vi "Bind Delete Command Parameters.vi"(8 "Error In (no error)":errorcluster, 10 "Record":variant, 11 "SQL Statement In":refnum<class "SQL Statement.lvclass">) -> (0 "Error Out":errorcluster, 3 "SQL Statement Out":refnum<class "SQL Statement.lvclass">)   [LabVIEW 2023, in "SQLite DB Operator.lvclass"]
uses:
  <vilib>/drjdpowell/SQLite Library/SQL Statement/SQL Statement.lvclass
  DB Records/Expenses Tracker Balance/Public/Ctrls/Balance.ctl
  <vilib>/drjdpowell/SQLite Library/SQL Statement/SQL Statement.lvclass/SQL Statement.ctl
  DB Records/Expenses Tracker Category/Public/Ctrls/Category.ctl
  DB Records/Expenses Tracker Cycle/Public/Ctrls/Cycle.ctl
  DB Records/Expenses Tracker Saving Goal/Public/Ctrls/Saving Goal.ctl
  DB Records/Expenses Tracker Saving/Public/Ctrls/Saving.ctl
  DB Records/Expenses Tracker Subcategory/Public/Ctrls/Subcategory.ctl
  DB Records/Expenses Tracker Transaction/Public/Ctrls/Transaction.ctl
  <vilib>/drjdpowell/SQLite Library/SQL Statement/Bind Null.vi
  <vilib>/drjdpowell/SQLite Library/SQL Statement/Bind Timestamp (Real).vi
  <vilib>/drjdpowell/SQLite Library/SQL Statement/Bind Real.vi
  <vilib>/drjdpowell/SQLite Library/SQL Statement/Bind Integer.vi
  <vilib>/drjdpowell/SQLite Library/SQL Statement/Bind Text.vi
  <vilib>/drjdpowell/SQLite Library/SQL Statement/Error Message.vi
  SQLite DB Operator.lvclass
  SQLite DB Operator.lvclass/SQLite DB Operator.ctl
  DB Records/Expenses Tracker Category/Expenses Tracker Category.lvclass
  <vilib>/Utility/Data Type/NI_Data Type.lvlib
  DB Records/Expenses Tracker Transaction/Expenses Tracker Transaction.lvclass
  DB Records/Expenses Tracker Subcategory/Expenses Tracker Subcategory.lvclass
  DB Records/Expenses Tracker Balance/Expenses Tracker Balance.lvclass
  DB Records/Expenses Tracker Cycle/Expenses Tracker Cycle.lvclass
  DB Records/Expenses Tracker Saving Goal/Expenses Tracker Saving Goal.lvclass
  DB Records/Expenses Tracker Saving/Expenses Tracker Saving.lvclass
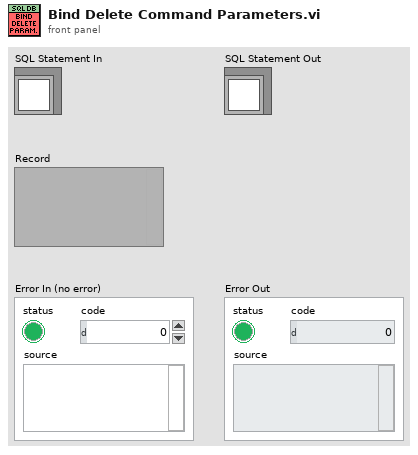
[diagram p1: front panel]
types:
  T1 = typedef "Expenses Tracker Balance.lvclass/Balance.ctl" = cluster{"ID":u8, "Value":dbl, "Last_update":timestamp}
  T2 = typedef "Expenses Tracker Category.lvclass/Category.ctl" = cluster{"ID":u32, "Name":string}
  T3 = typedef "Expenses Tracker Cycle.lvclass/Cycle.ctl" = cluster{"ID":u32, "Name":string, "Day_of_occurence":u8, "Description":string}
  T4 = typedef "Expenses Tracker Saving Goal.lvclass/Saving Goal.ctl" = cluster{"ID":u32, "Name":string, "Current_value":dbl, "Target_value":dbl, "Date_of_entry":timestamp, "Due_date":timestamp, "Last_update":timestamp, "Description":string}
  T5 = typedef "Expenses Tracker Saving.lvclass/Saving.ctl" = cluster{"ID":u32, "Saving_goal":u32, "Value":dbl, "Date_of_entry":timestamp, "Description":string}
  T6 = typedef "Expenses Tracker Subcategory.lvclass/Subcategory.ctl" = cluster{"ID":u32, "Name":string, "Category":u32}
  T7 = typedef "Expenses Tracker Transaction.lvclass/Transaction.ctl" = cluster{"ID":u32, "Name":string, "Is_income":bool, "Value":dbl, "Amount":dbl, "Total":dbl, "Date_of_entry":timestamp, "Date_of_occurence":timestamp, "Last_update":timestamp, "Category":u32, "Subcategory":u32, "Cycle":u32, "Description":string}
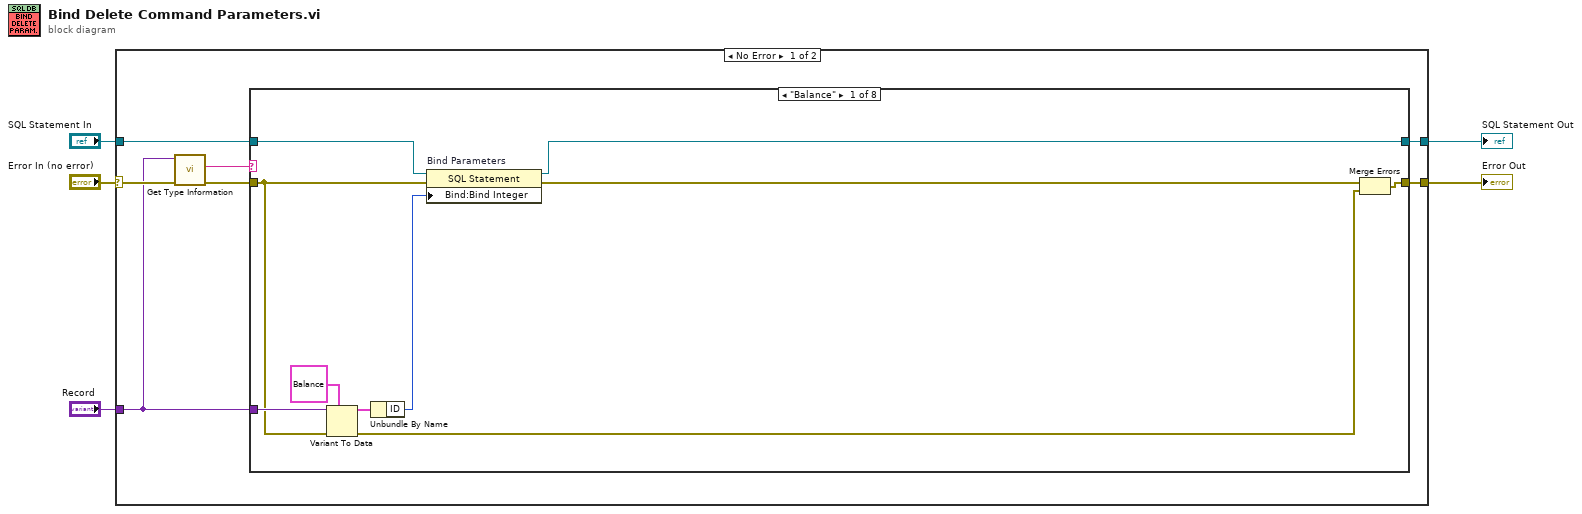
[diagram p0: block diagram]
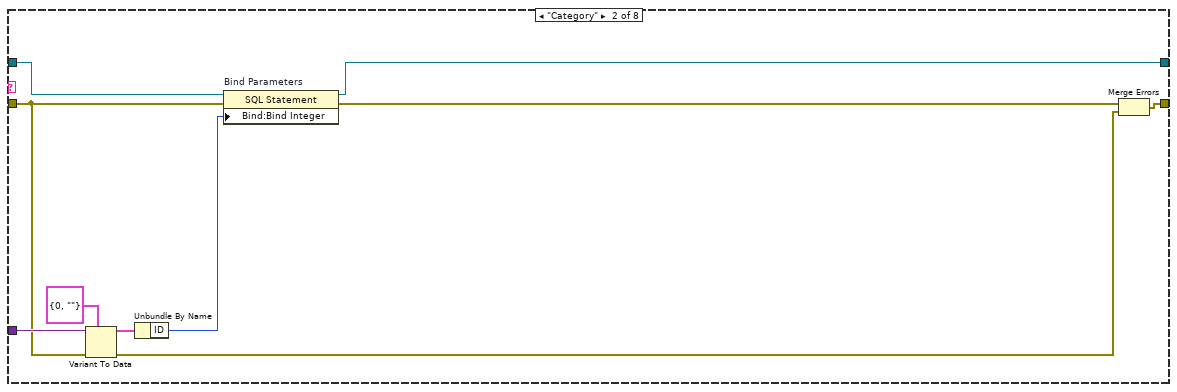
[diagram p2: hidden frame]
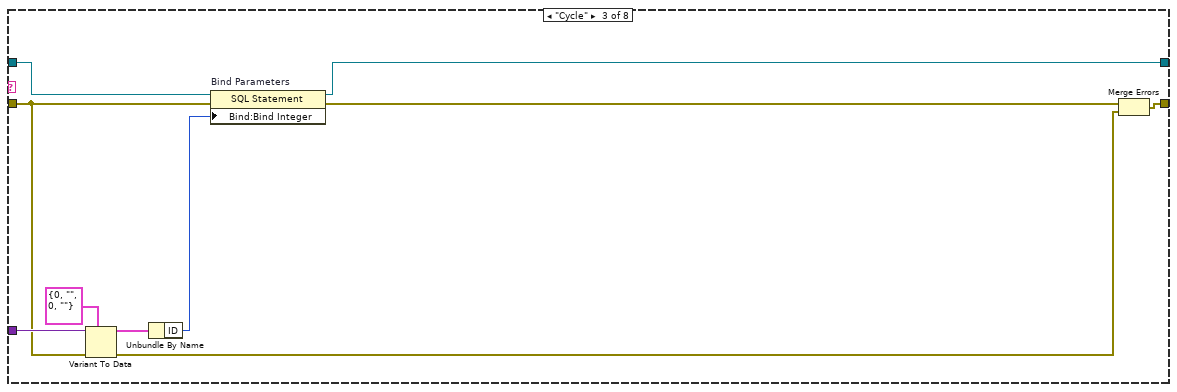
[diagram p3: hidden frame]
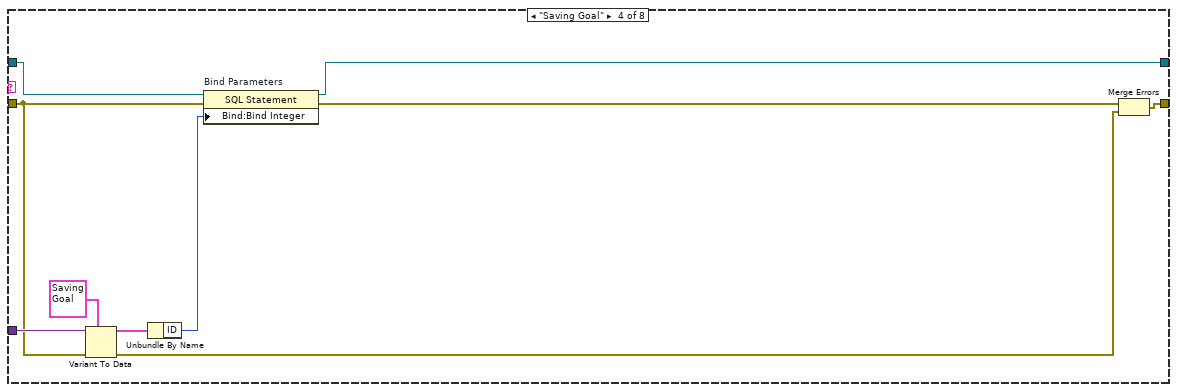
[diagram p4: hidden frame]
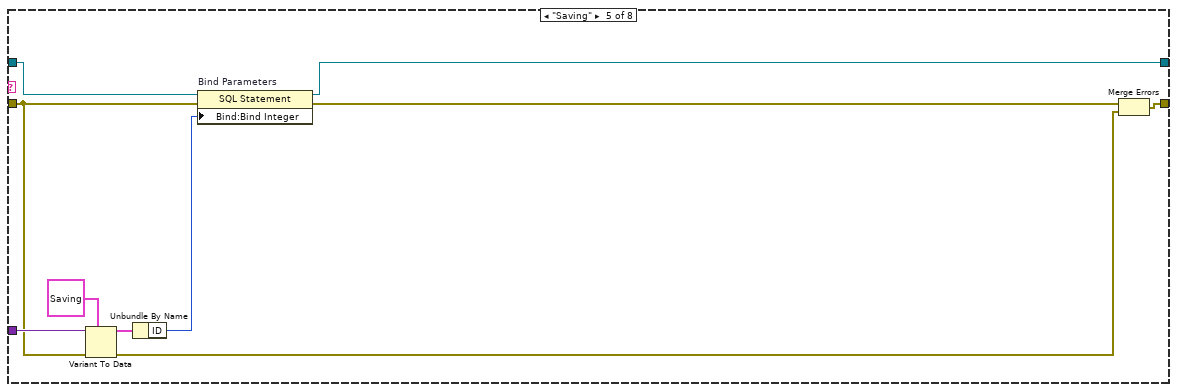
[diagram p5: hidden frame]
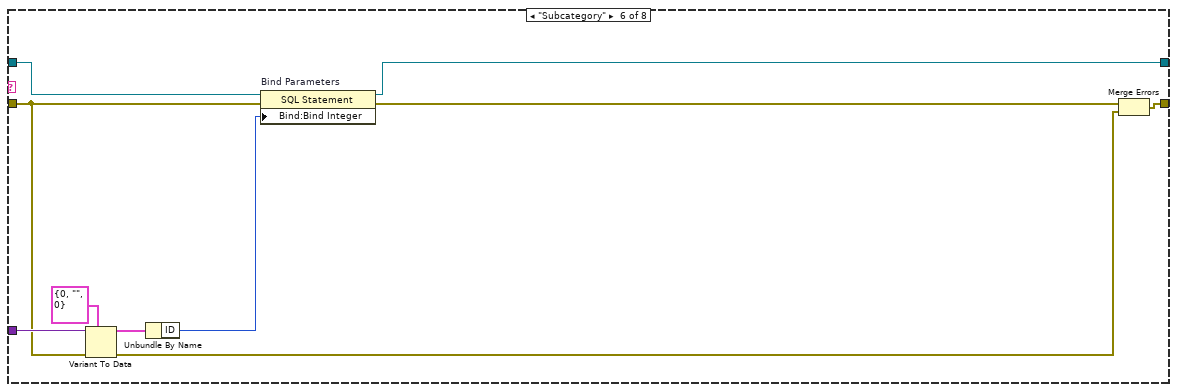
[diagram p6: hidden frame]
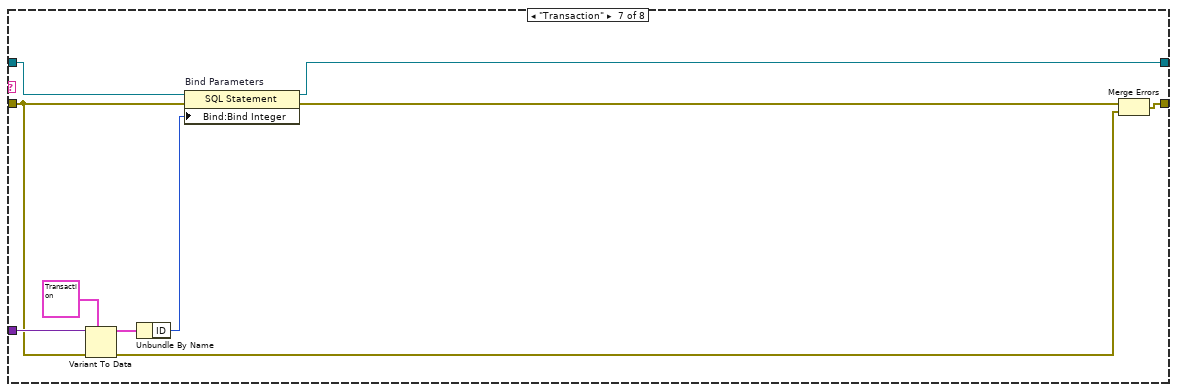
[diagram p7: hidden frame]
diagram:
  n1 = case shown="No Error" "Error In (no error)" {
    selector: "Error In (no error)" -> [w9 w85]
    tunnel: "SQL Statement In" -> [w12 w86]
    tunnel: [w11 w85] -> w4
    tunnel: [w10 w86] -> w3
    tunnel: "Record" -> [w8 _]
    frame No Error {
      n2 = call <vilib>:"Get Type Information.vi"("error in (no error)"=w9, "variant"=w8) -> ("error out"=w6:errorcluster, "name"=w7:string)  [unwired: 5 in, 3 out]
      n3 = case shown="\"Balance\"" w7 {
        tunnel: w8 -> [w22 w32 w42 w52 w62 w72 w82 _]
        tunnel: [w15 w31 w34 w46 w56 w71 w76 w84] -> w10
        tunnel: [w19 w27 w39 w49 w59 w67 w79 w83] -> w11
        tunnel: w12 -> [w16 w24 w36 w44 w54 w64 w74 w84]
        tunnel: w6 -> [w17 w25 w37 w45 w55 w65 w75 w83]
        frame "Balance" {
          n4 = Variant To Data(error in=w17, type=T1 {"ID"=0, "Value"=0.0, "Last_update"=timestamp(0 s since 1904-01-01)} ("Balance"), Variant=w22) -> (data=w21:T1, error out=w18:errorcluster)
          n5 = Unbundle By Name(w21) -> ("ID"=w13:u8)
          n6 = property on="Bind Parameters" class="SQL Statement"(reference=w16, error in=w17, "Bind:Bind Integer"=w13) -> (reference out=w15:refnum<class "SQL Statement.lvclass">, error out=w14:errorcluster)
          n7 = Merge Errors(w14, w18) -> (w19:errorcluster)
        }
        frame "Category" {
          n8 = Variant To Data(error in=w25, type=T2 {"ID"=0, "Name"=""} ("Category"), Variant=w32) -> (data=w29:T2, error out=w26:errorcluster)
          n9 = Unbundle By Name(w29) -> ("ID"=w23:u32)
          n10 = property on="Bind Parameters" class="SQL Statement"(reference=w24, error in=w25, "Bind:Bind Integer"=w23) -> (reference out=w31:refnum<class "SQL Statement.lvclass">, error out=w30:errorcluster)
          n11 = Merge Errors(w30, w26) -> (w27:errorcluster)
        }
        frame "Cycle" {
          n12 = Variant To Data(error in=w37, type=T3 {"ID"=0, "Name"="", "Day_of_occurence"=0, "Description"=""} ("Cycle"), Variant=w42) -> (data=w41:T3, error out=w38:errorcluster)
          n13 = Unbundle By Name(w41) -> ("ID"=w33:u32)
          n14 = property on="Bind Parameters" class="SQL Statement"(reference=w36, error in=w37, "Bind:Bind Integer"=w33) -> (reference out=w34:refnum<class "SQL Statement.lvclass">, error out=w35:errorcluster)
          n15 = Merge Errors(w35, w38) -> (w39:errorcluster)
        }
        frame "Saving Goal" {
          n16 = Variant To Data(error in=w45, type=T4 {"ID"=0, "Name"="", "Current_value"=0.0, "Target_value"=0.0, "Date_of_entry"=timestamp(0 s since 1904-01-01), "Due_date"=timestamp(0 s since 1904-01-01), "Last_update"=timestamp(0 s since 1904-01-01), "Description"=""} ("Saving Goal"), Variant=w52) -> (data=w51:T4, error out=w48:errorcluster)
          n17 = Unbundle By Name(w51) -> ("ID"=w43:u32)
          n18 = property on="Bind Parameters" class="SQL Statement"(reference=w44, error in=w45, "Bind:Bind Integer"=w43) -> (reference out=w46:refnum<class "SQL Statement.lvclass">, error out=w47:errorcluster)
          n19 = Merge Errors(w47, w48) -> (w49:errorcluster)
        }
        frame "Saving" {
          n20 = Variant To Data(error in=w55, type=T5 {"ID"=0, "Saving_goal"=0, "Value"=0.0, "Date_of_entry"=timestamp(0 s since 1904-01-01), "Description"=""} ("Saving"), Variant=w62) -> (data=w61:T5, error out=w58:errorcluster)
          n21 = Unbundle By Name(w61) -> ("ID"=w53:u32)
          n22 = property on="Bind Parameters" class="SQL Statement"(reference=w54, error in=w55, "Bind:Bind Integer"=w53) -> (reference out=w56:refnum<class "SQL Statement.lvclass">, error out=w57:errorcluster)
          n23 = Merge Errors(w57, w58) -> (w59:errorcluster)
        }
        frame "Subcategory" {
          n24 = Variant To Data(error in=w65, type=T6 {"ID"=0, "Name"="", "Category"=0} ("Subcategory"), Variant=w72) -> (data=w69:T6, error out=w66:errorcluster)
          n25 = Unbundle By Name(w69) -> ("ID"=w63:u32)
          n26 = property on="Bind Parameters" class="SQL Statement"(reference=w64, error in=w65, "Bind:Bind Integer"=w63) -> (reference out=w71:refnum<class "SQL Statement.lvclass">, error out=w70:errorcluster)
          n27 = Merge Errors(w70, w66) -> (w67:errorcluster)
        }
        frame "Transaction" {
          n28 = Variant To Data(error in=w75, type=T7 {"ID"=0, "Name"="", "Is_income"=FALSE, "Value"=0.0, "Amount"=0.0, "Total"=0.0, "Date_of_entry"=timestamp(0 s since 1904-01-01), "Date_of_occurence"=timestamp(0 s since 1904-01-01), "Last_update"=timestamp(0 s since 1904-01-01), "Category"=0, "Subcategory"=0, "Cycle"=0, "Description"=""} ("Transaction"), Variant=w82) -> (data=w81:T7, error out=w78:errorcluster)
          n29 = Unbundle By Name(w81) -> ("ID"=w73:u32)
          n30 = property on="Bind Parameters" class="SQL Statement"(reference=w74, error in=w75, "Bind:Bind Integer"=w73) -> (reference out=w76:refnum<class "SQL Statement.lvclass">, error out=w77:errorcluster)
          n31 = Merge Errors(w77, w78) -> (w79:errorcluster)
        }
        frame Default {
        }
      }
    }
    frame Error {
    }
  }
  "Error Out" <- w4
  "SQL Statement Out" <- w3
